vi "CloseCollector.vi"(8 "error in (no error)":errorcluster, 11 "DataCollector in":refnum<class "DataCollector.lvclass">) -> (0 "error out":errorcluster, 3 "DataCollector out":refnum<class "DataCollector.lvclass">)   [LabVIEW 2017, in "DataCollector.lvclass"]
uses:
  DataCollector.lvclass
  DataCollector.lvclass/DataCollector.ctl
  <vilib>/drjdpowell/SQLite Library/SQL Connection/Connection.lvclass
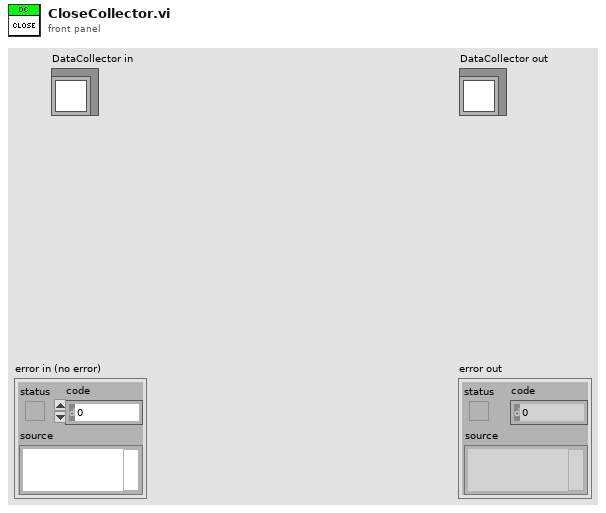
[diagram p1: front panel]
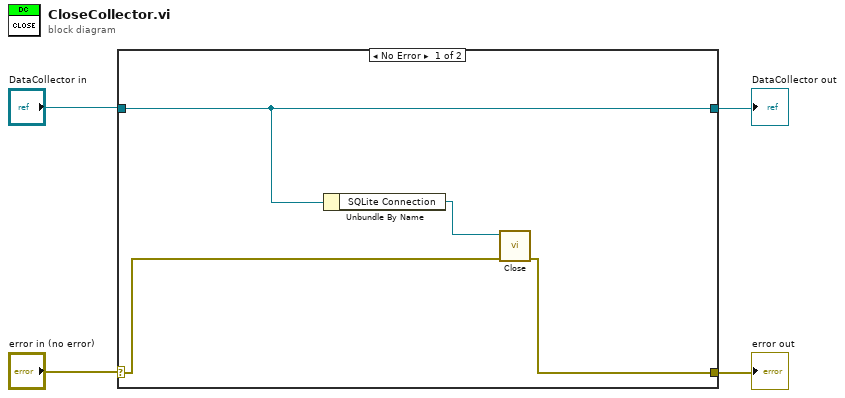
[diagram p0: block diagram]
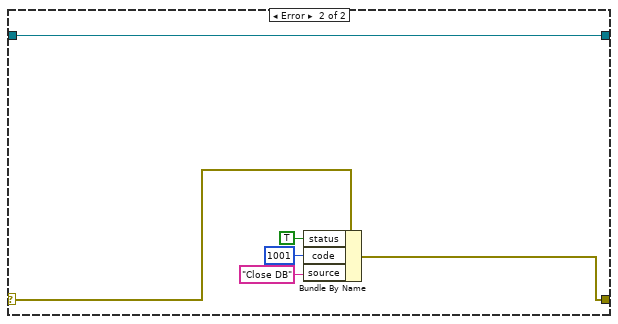
[diagram p2: hidden frame]
diagram:
  n1 = case shown="No Error" "error in (no error)" {
    selector: "error in (no error)" -> [w6 w13]
    tunnel: [w5 w12] -> w1
    tunnel: [w7 w14] -> w3
    tunnel: "DataCollector in" -> [w7 w14]
    frame No Error {
      n2 = Unbundle By Name(w7) -> ("SQLite Connection"=w8:refnum<class "Connection.lvclass">)
      n3 = call-dynamic "Close.vi"("error in (no error)"=w6, "SQLite Connection in"=w8) -> ("error out"=w5:errorcluster)  [unwired: 9 in]
    }
    frame Error {
      n4 = Bundle By Name(cluster=w13, "status"=TRUE, "code"=1001, "source"="Close DB") -> (w12:errorcluster)
    }
  }
  "error out" <- w1
  "DataCollector out" <- w3
